vi "Initialize Cache.vi"(8 "error in (no error)":errorcluster, 9 "Initialized Array in":bool[](array[boolean]), 10 "Array in":waveform(dbl)[](array[waveform]), 11 "Current Cache in":T1[](array[typedef])) -> (0 "error out":errorcluster, 3 "Current Cache out":T1[](array[typedef]))   [LabVIEW 2026, in "Processing_Engine.lvlib"]
uses:
  Processing_Engine.lvlib
  controls/Messaging Payloads/Processed Calibration Point.ctl
  controls/UI/Direction.ctl
  Test Status.ctl
  Analysis/Analysis.lvlib
  Settings/Settings.lvlib
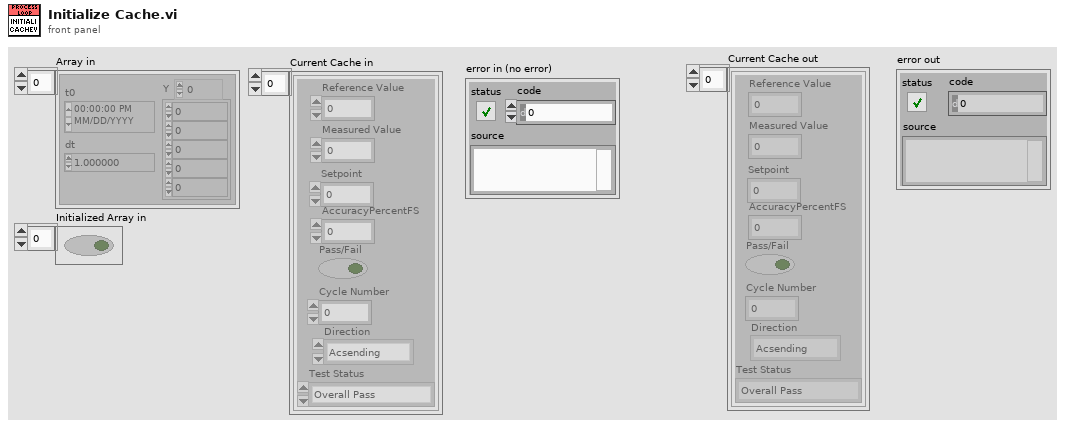
[diagram p1: front panel]
types:
  T1 = typedef "Processed Calibration Point.ctl" = cluster{"Reference Value":dbl, "Measured Value":dbl, "AccuracyPercentFS":dbl, "Pass/Fail":bool, "Setpoint":dbl, "Cycle Number":i32, "Direction":T2, "Test Status":T3}
  T2 = typedef "Settings.lvlib/Direction.ctl" = enum16{"Acsending", "Descending"}
  T3 = typedef "Analysis.lvlib/Test Status.ctl" = enum16{"Overall Pass", "Overall Fail", "Test Running"}
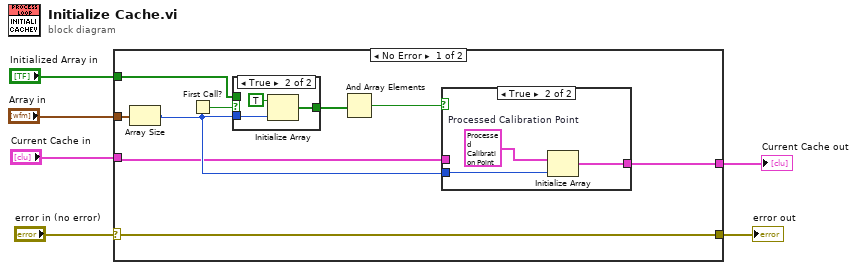
[diagram p0: block diagram]
diagram:
  n1 = case shown="No Error" "error in (no error)" {
    selector: "error in (no error)" -> [w9 w25]
    tunnel: "Initialized Array in" -> [w14 _]
    tunnel: [w12 w24] -> w5
    tunnel: "Array in" -> [w11 _]
    tunnel: [w9 w25] -> w2
    tunnel: "Current Cache in" -> [w8 w24]
    frame No Error {
      n2 = Array Size(array=w11) -> (size(s)=w10:i32)
      n3 = First Call?() -> (First Call?: T/F=w15:bool)
      n4 = case shown="True" w15 {
        tunnel: w10 -> [_ w22]
        tunnel: [w20 w21] -> w13
        tunnel: w14 -> [w20 _]
        frame False {
        }
        frame True {
          n5 = Initialize Array(TRUE ("Record?"), w22) -> (w21:bool[])
        }
      }
      n6 = And Array Elements(Boolean array=w13) -> (logical AND=w7:bool)
      n7 = case shown="True" w7 {
        tunnel: w10 -> [_ w18]
        tunnel: [w16 w17] -> w12
        tunnel: w8 -> [w16 _]
        frame False {
        }
        frame True {
          w19 = T1 {"Reference Value"=0.0, "Measured Value"=0.0, "AccuracyPercentFS"=0.0, "Pass/Fail"=TRUE, "Setpoint"=0.0, "Cycle Number"=0, "Direction"=enum."Acsending", "Test Status"=enum."Overall Fail"}  # Processed Calibration Point
          n8 = Initialize Array(w19, w18) -> (w17:T1[])
        }
      }
    }
    frame Error {
    }
  }
  "error out" <- w2
  "Current Cache out" <- w5
